vi "computeHashToRange.vi"(8 "min Value":i32, 10 "maxValue":i32=59, 11 "seed":string) -> (1 "H":i32)   [LabVIEW 2013, in "openCron.lvlib" / "Cron.lvclass"]
uses:
  Cron.lvclass
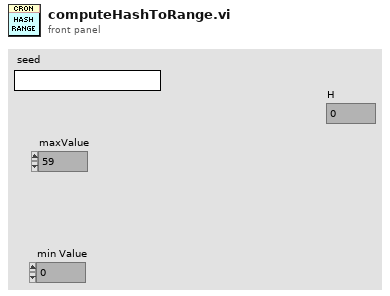
[diagram p1: front panel]
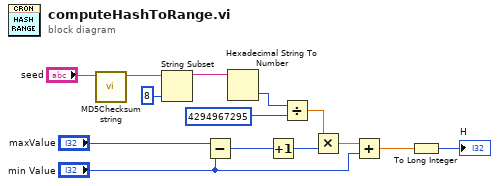
[diagram p0: block diagram]
diagram:
  n1 = call <vilib>:"MD5Checksum string.vi"("Message String"="seed") -> ("MD5 message-digest"=w5:string)  [unwired: 10 in]
  n2 = String Subset(string=w5, length (rest)=i16 8 ("width (-)")) -> (substring=w3:string)  [unwired: 1 in]
  n3 = Subtract(x="maxValue", y="min Value") -> (x-y=w9:i32)
  n4 = Hexadecimal String To Number(string=w3) -> (number=w2:u32)  [unwired: 2 in, 1 out]
  n5 = Increment(x=w9) -> (x+1=w8:i32)
  n6 = Divide(x=w2, y=u32 4294967295) -> (x/y=w6:dbl)
  n7 = Multiply(x=w6, y=w8) -> (x*y=w7:dbl)
  n8 = Add(x=w7, y="min Value") -> (x+y=w11:dbl)
  n9 = To Long Integer(number=w11) -> (32bit integer=→"H":i32)
